vi "StartDLControlVI.vi"(8 "entrée d'erreur (pas d'erreur)":errorcluster, 11 "Control en entrée":refnum<class "Control-Server.lvclass">) -> (0 "sortie d'erreur":errorcluster, 3 "Control en sortie":refnum<class "Control-Server.lvclass">)   [LabVIEW 2015, in "Control-Server.lvclass"]
uses:
  Classes/Control/Control-Server/Control-Server.lvclass
  Classes/Control/Control-Server/Control-Server.lvclass/Control-Server.ctl
  Clusters-def/Message types.ctl
  Classes/Message/Message.lvclass/Message.ctl
  Classes/Delay Line/DelayLine.lvclass
  Classes/Message/Message.lvclass
  Classes/GeneralFunctionality/GeneralFunctionality.lvclass
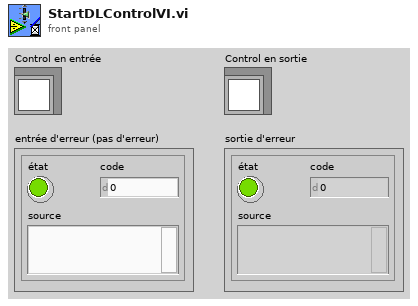
[diagram p1: front panel]
types:
  T1 = typedef "Message types.ctl" = string
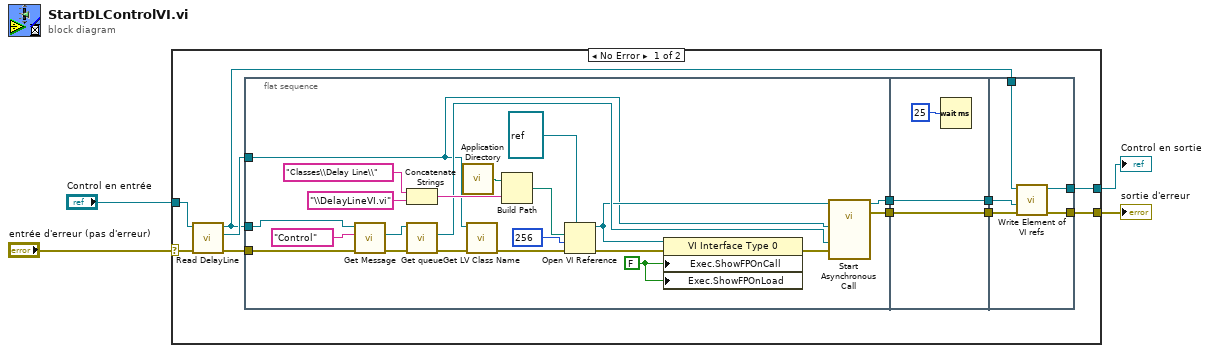
[diagram p0: block diagram]
diagram:
  n1 = case shown="No Error" "entrée d'erreur (pas d'erreur)" {
    selector: "entrée d'erreur (pas d'erreur)" -> [w11 w47]
    tunnel: [w15 w47] -> w4
    tunnel: "Control en entrée" -> [w14 w46]
    tunnel: [w9 w46] -> w2
    frame No Error {
      n2 = call "Read DelayLine.vi"("error in (no error)"=w11, "Control in"=w14) -> ("error out"=w12:errorcluster, "DelayLine.lvclass"=w13:refnum<class "DelayLine.lvclass">, "Control out"=w10:refnum<class "Control-Server.lvclass">)  [unwired: 7 in]
      n3 = flat-sequence {
        tunnel: [w24] -> w8
        tunnel: w13 -> [w17]
        tunnel: [w23] -> w6
        tunnel: w12 -> [w26]
        tunnel: w10 -> [w27]
        tunnel: w8 -> [w40]
        tunnel: [w40] -> w7
        tunnel: w6 -> [w39]
        tunnel: [w39] -> w5
        tunnel: [w42] -> w15
        tunnel: w7 -> [w41]
        tunnel: w10 -> [w43]
        tunnel: [w45] -> w9
        tunnel: w5 -> [w44]
        frame #0 {
          w31 = FALSE ("Execution:Show Front Panel On Call")
          n4 = call "Get Message.vi"("error in (no error)"=w26, "Message type"=T1 "Control", "GeneralFunctionality en entrée"=w27) -> ("error out"=w20:errorcluster, "Message.lvclass"=w21:refnum<class "Message.lvclass">)  [unwired: 6 in, 1 out]
          n5 = Concatenate Strings("Classes\\Delay Line\\" ("chaîne"), "\\DelayLineVI.vi" ("chaîne")) -> (w30:string)
          n6 = call "Get queue.vi"("error in (no error)"=w20, "Message in"=w21) -> ("error out"=w16:errorcluster, "queue"=w19:refnum<queue>)  [unwired: 7 in, 1 out]
          n7 = call <vilib>:"Application Directory.vi"() -> ("Application Directory"=w35:path)
          n8 = call <vilib>:"Get LV Class Name.vi"("error in (no error)"=w16, "object"=w17) -> ("error out"=w37:errorcluster)  [unwired: 8 in, 1 out]
          n9 = Build Path(base path=w35, name or relative path=w30) -> (appended path=w36:path)
          n10 = Open VI Reference(type specifier VI Refnum (for type only)=refnum<vi> refnum ("spécificateur de type du refnum de VI (pour type seulement)"), vi path=w36, options=256, error in (no error)=w37) -> (vi reference=w18:refnum<vi>, error out=w32:errorcluster)  [unwired: 2 in]
          n11 = property class="VI Interface Type 0"(reference=w18, error in=w32, "Exec.ShowFPOnCall"=w31, "Exec.ShowFPOnLoad"=w31) -> (error out=w22:errorcluster)  [unwired: 1 out]
          n12 = call-by-ref "Start Asynchronous Call"(reference=w18, "error in (no error)"=w22, "ControlQueue"=w19, "DelayLine.lvclass"=w17) -> (reference out=w23:refnum<vi>, error out=w24:errorcluster)  [unwired: 9 in, 1 out]
        }
        frame #1 {
          n13 = Wait (ms)(milliseconds to wait=u32 25) -> ()  [unwired: 1 out]
        }
        frame #2 {
          n14 = call "Write Element of VI refs.vi"("error in (no error)"=w41, "vi reference"=w44, "Control in"=w43) -> ("error out"=w42:errorcluster, "Control out"=w45:refnum<class "Control-Server.lvclass">)  [unwired: 7 in]
        }
      }
    }
    frame Error {
    }
  }
  "sortie d'erreur" <- w4
  "Control en sortie" <- w2
